vi "Abbreviate Classes in Library.vi"(10 "Abbreviate Name?":bool, 11 "Name":string) -> (3 "Name out":string)   [LabVIEW 2020, in "VI Properties Editor.lvlib"]
doc: "Abbreviates a VI name if the VI is in a class which itself is in a library."
uses:
  VI Properties Editor.lvlib
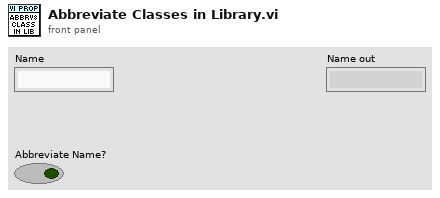
[diagram p1: front panel]
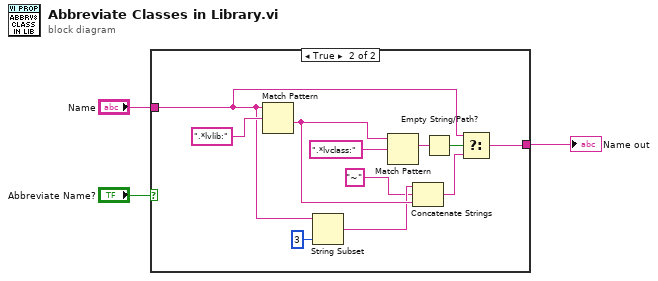
[diagram p0: block diagram]
diagram:
  n1 = case shown="True" "Abbreviate Name?" {
    tunnel: "Name" -> [w4 w9]
    tunnel: [w4 w15] -> w2
    frame False {
    }
    frame True {
      n2 = Match Pattern(string=w9, regular expression=".*lvlib:") -> (after substring=w10:string)  [unwired: 1 in, 3 out]
      n3 = String Subset(string=w9, length (rest)=3 ("length (rest)")) -> (substring=w6:string)  [unwired: 1 in]
      n4 = Match Pattern(string=w10, regular expression=".*lvclass:") -> (match substring=w12:string)  [unwired: 1 in, 3 out]
      n5 = Concatenate Strings(w6, "~" ("string"), w10) -> (w7:string)
      n6 = Empty String/Path?(string/path=w12) -> (empty?=w11:bool)
      n7 = Select(t=w9, s=w11, f=w7) -> (s? t:f=w15:string)
    }
  }
  "Name out" <- w2
